vi "Receive Datum Update.vi"(8 "Publication Time":timestamp, 9 "Value":variant, 10 "Datum Name":string, 11 "ListboxBusMonitorPanel in":refnum<class "ListboxBusMonitorPanel.lvclass">) -> (3 "ListboxBusMonitorPanel out":refnum<class "ListboxBusMonitorPanel.lvclass">)   [LabVIEW 2019, in "ListboxBusMonitor.lvlib" / "ListboxBusMonitorPanel.lvclass"]
uses:
  <vilib>/gpm_packages/@cs/BusMonitor/ListboxBusMonitor/ListboxBusMonitorPanel/ListboxBusMonitorPanel.lvclass
  <vilib>/gpm_packages/@cs/BusMonitor/ListboxBusMonitor/ListboxBusMonitorPanel/ListboxBusMonitorPanel.lvclass/ListboxBusMonitorPanel.ctl
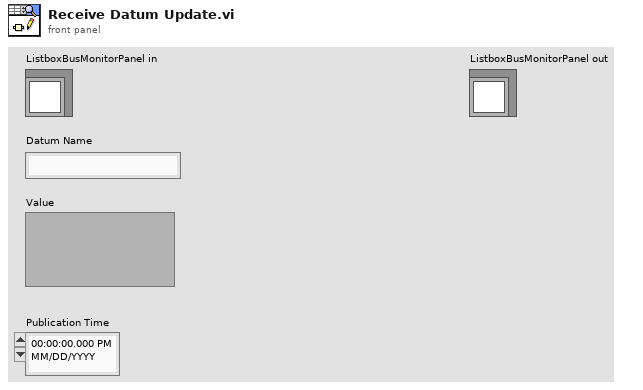
[diagram p1: front panel]
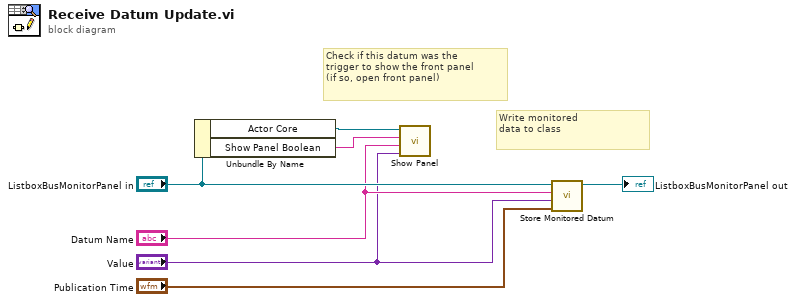
[diagram p0: block diagram]
diagram:
  # "Write monitored\ndata to class"
  # "Check if this datum was the\ntrigger to show the front panel\n(if so, open front panel)"
  n1 = Unbundle By Name("ListboxBusMonitorPanel in") -> ("Actor Core"=w7:refnum<vi>, "Show Panel Boolean"=w4:string)
  n2 = call <vilib>:"Show Panel.vi"("Value"="Value", "Datum Name"="Datum Name", "Show Panel Boolean"=w4, "VI in"=w7) -> ()  [unwired: 8 in]
  n3 = call <vilib>:"Store Monitored Datum.vi"("Publication Time"="Publication Time", "Value"="Value", "Datum Name"="Datum Name", "ListboxBusMonitorPanel in"="ListboxBusMonitorPanel in") -> ("ListboxBusMonitorPanel out"=→"ListboxBusMonitorPanel out":refnum<class "ListboxBusMonitorPanel.lvclass">)  [unwired: 7 in]
